vi "Setup UI.vi"(8 "error in (no error)":errorcluster, 10 "Set UI to input? (F)":bool, 11 "Pulse Gen Scan in":refnum<class "Pulse Gen Scan.lvclass">) -> (0 "error out":errorcluster, 3 "Pulse Gen Scan out":refnum<class "Pulse Gen Scan.lvclass">)   [LabVIEW 2015, in "Pulse Gen Scan.lvclass"]
doc: "Scanner::Setup is a constructor that has no parameters and faces the user. The Factory calls this VI to let the user configure this Scanner. It is dynamically dispatched in order to let the user choose the type as well as the options of the scanner."
uses:
  Pulse Gen Scan.lvclass
  Pulse Gen Scan.lvclass/Pulse Gen Scan.ctl
panel:
  in  "Gated":bool
  in  "Switch Ch1 and Ch2 Outputs":bool
  in  "template: seperate \nch 1 pump/ ch2 probe":bool
  in  "Width/Dutycycle\nUP/Down":bool
  in  "dutycycle3":dbl
  in  "dutycycle2":dbl
  in  "dutycycle1":dbl
  out "Expected external period/frequency (text)":string="Expected external period/frequency"
  out "Desired overall period/frequency (text)":string="Desired overall period/frequency"
  in  "Trigger Mode":bool caption="External"
  in  "template: Rabi scan":bool
  out "Array of Ch2 times used":dbl[unit][](array[numeric])
  in  "Repeat sequence,\ncentered on 3T/4?":bool
  in  "Ch1 pulses centered \non trigger T/4?":enum32{"none", "first", "second"}(radio)
  out "time per bit":dbl[unit]
  out "Array of Ch1 times used":dbl[unit][](array[numeric])
  in  "period/frequency":bool
  in  "template: spin echo scan":bool
  in  "template: pump/probe scan":bool
  in  "template: pulse width scan":bool
  in  "indCh2width?":bool
  in  "indChdelay?":bool
  in  "indWidth3?":bool
  in  "indDelay3?":bool
  in  "ind3Width2?":bool
  in  "indDelay2?":bool
  in  "indWidth1?":bool
  in  "indDelay1?":bool
  in  "Overall frequency":dbl[unit]
  in  "Overall period":dbl[unit]
  in  "Ch2width":dbl[unit]
  in  "Ch2delay":dbl[unit]
  in  "width3":dbl[unit]
  in  "delay3":dbl[unit]
  in  "width2":dbl[unit]
  in  "delay2":dbl[unit]
  in  "width1":dbl[unit]
  in  "delay1":dbl[unit]
  in  "Send conds for first point to PG":bool
  out "Ch 1 Digital Waveform Graph":digitalwaveform(graph)
  out "Ch1 output string":string
  out "Ch2 output string":string
  out "Ch 2 Digital Waveform Graph":digitalwaveform(graph)
  in  "Ch2 Delay relative \nto end of Ch1?":bool
  # "ind. variable?"
  # "PURE VIRTUAL\nMETHOD CALLED!"
  # "Internal"
  # "Pulse Gen Scan"
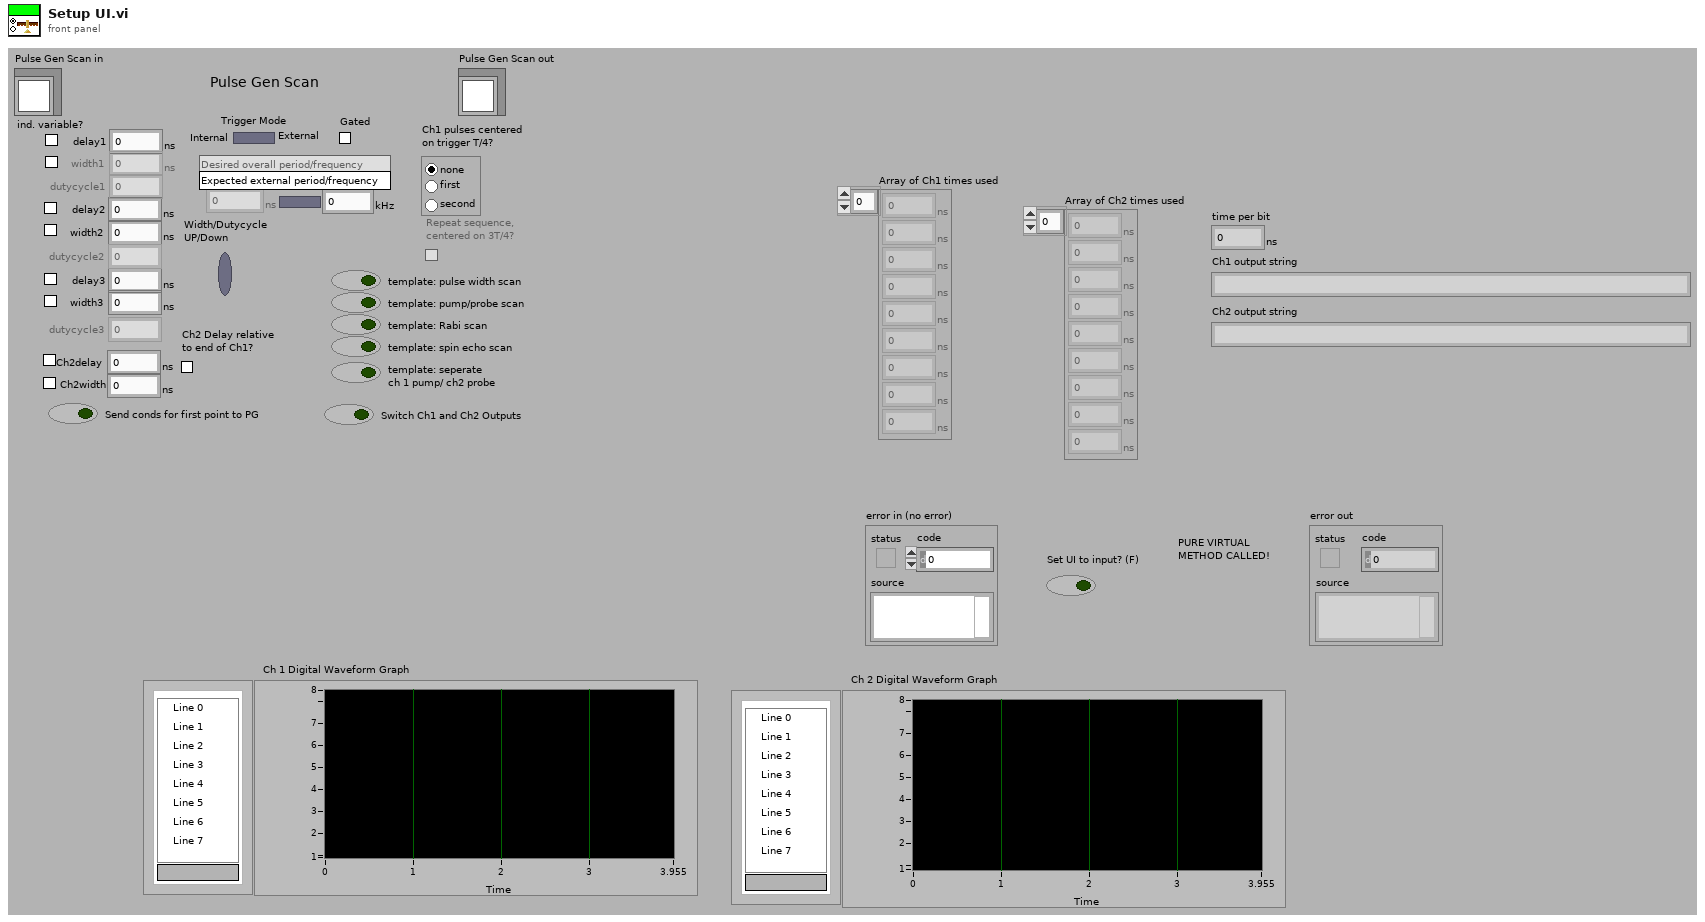
[diagram p1: front panel]
types:
  T1 = typedef "Scanner.lvclass/Range.ctl" = cluster{"xi":dbl, "xf":dbl, "dx":dbl, "Return to...?":bool, "Return to":dbl}
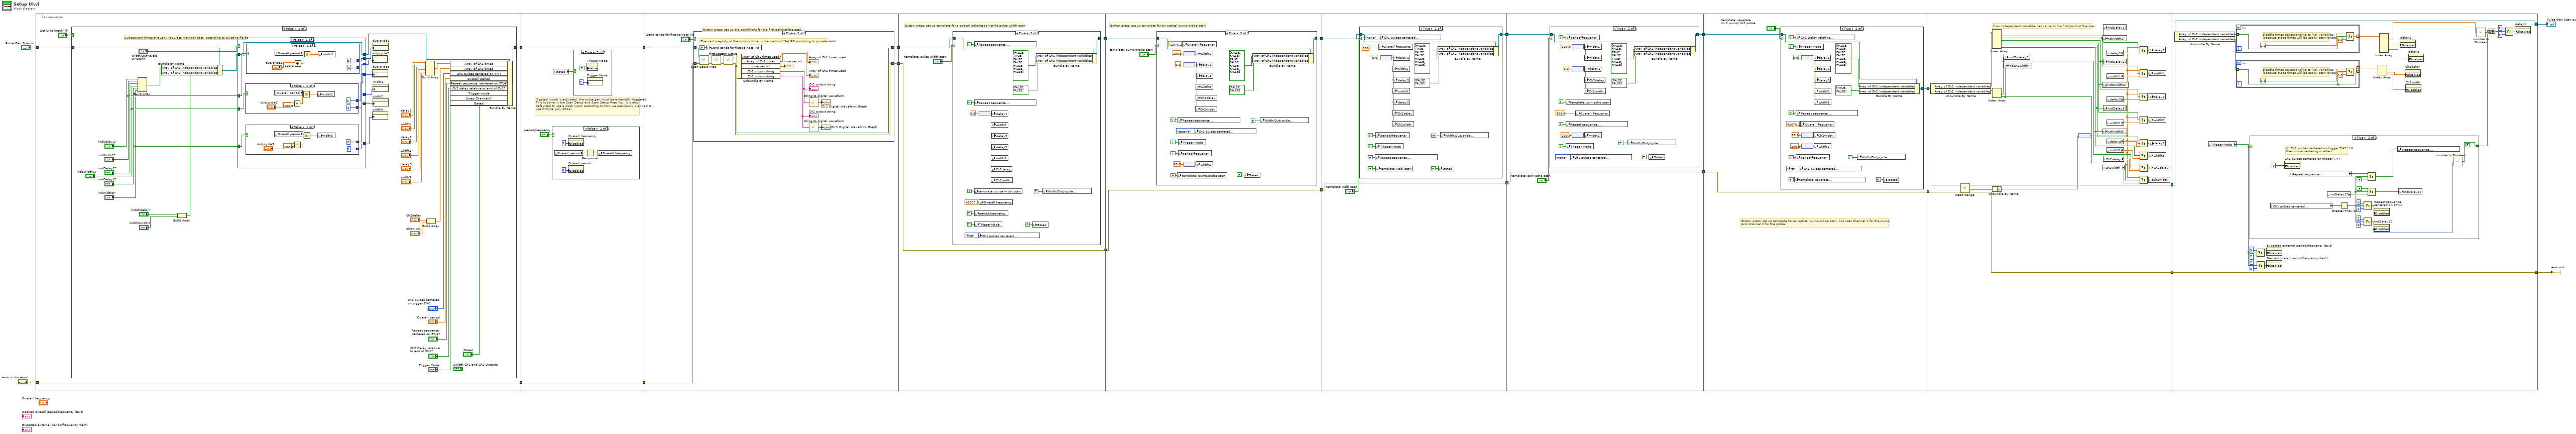
[diagram p0: block diagram]
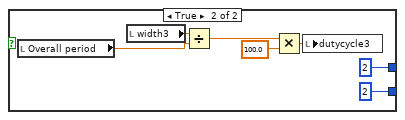
[diagram p2: hidden frame]
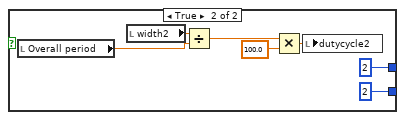
[diagram p3: hidden frame]
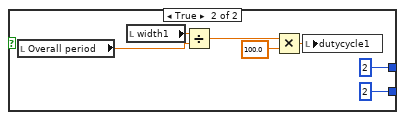
[diagram p4: hidden frame]
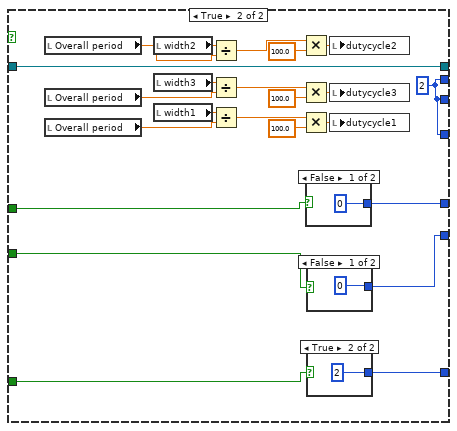
[diagram p5: hidden frame]
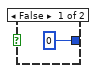
[diagram p6: hidden frame]
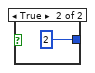
[diagram p7: hidden frame]
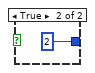
[diagram p8: hidden frame]
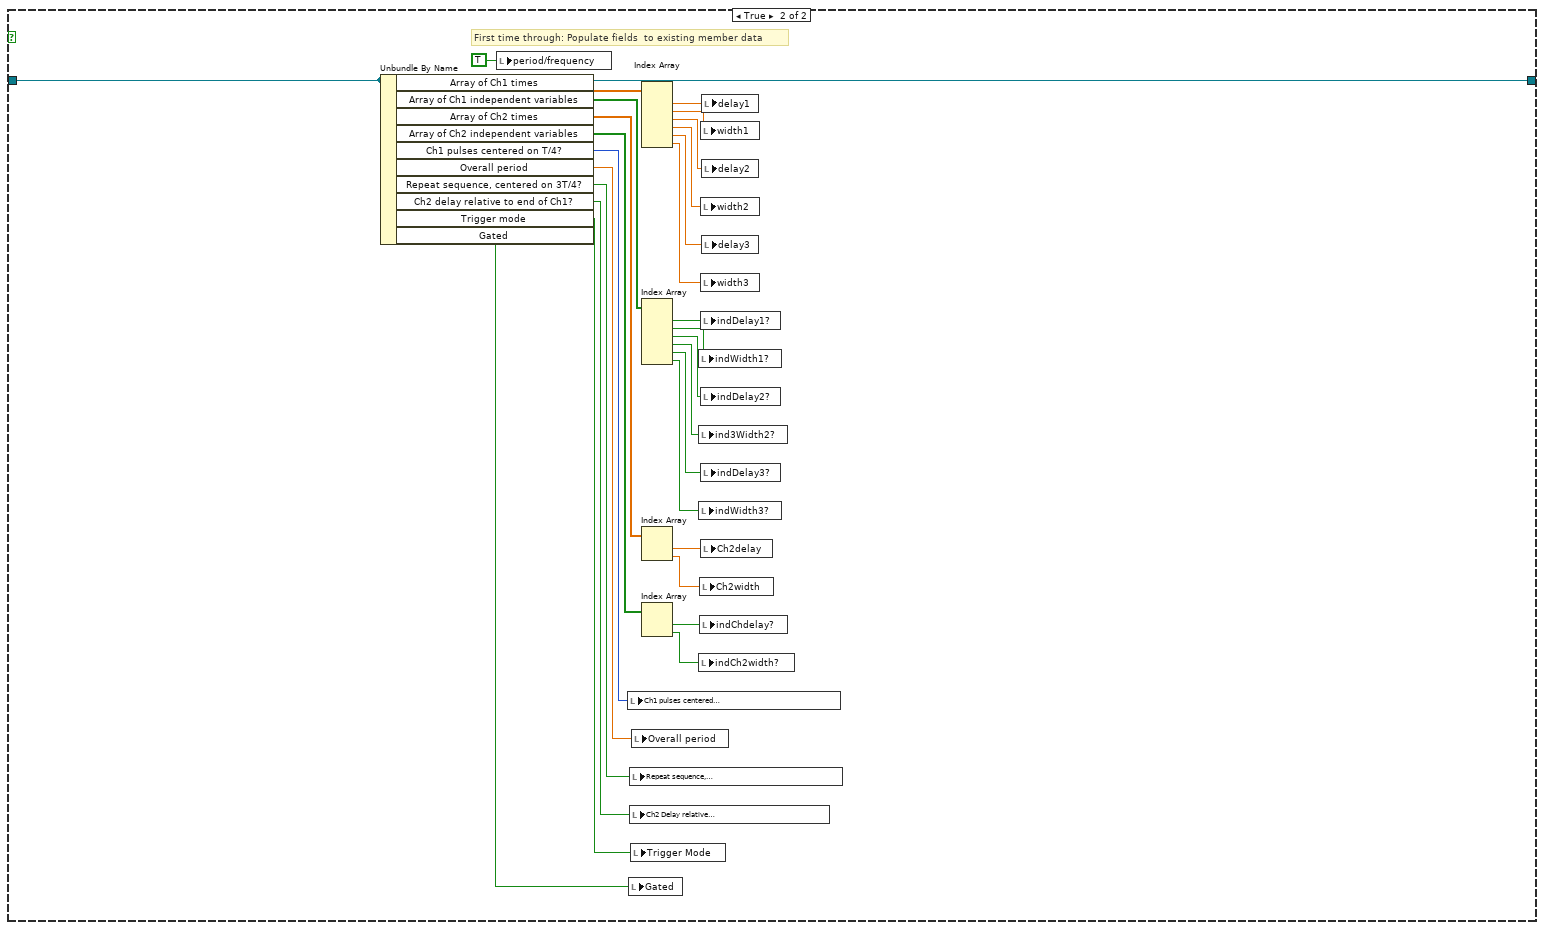
[diagram p9: hidden frame]
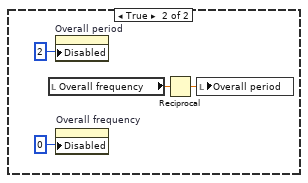
[diagram p10: hidden frame]
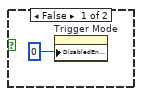
[diagram p11: hidden frame]
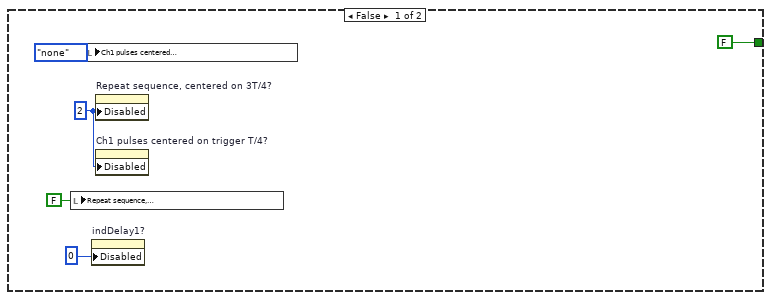
[diagram p18: hidden frame]
diagram:
  n1 = flat-sequence {
    tunnel: "error in (no error)" -> [w24]
    tunnel: "Pulse Gen Scan in" -> [w25]
    tunnel: [w23] -> w6
    tunnel: [w24] -> w4
    tunnel: w6 -> [w177]
    tunnel: [w177] -> w5
    tunnel: w4 -> [w176]
    tunnel: [w176] -> w3
    tunnel: w5 -> [w193]
    tunnel: [w191] -> w18
    tunnel: w3 -> [w192]
    tunnel: [w190] -> w17
    tunnel: w18 -> [w213]
    tunnel: [w214] -> w22
    tunnel: [w212] -> w21
    tunnel: w17 -> [w214]
    tunnel: [w232] -> w15
    tunnel: [w234] -> w13
    tunnel: w22 -> [w234]
    tunnel: w21 -> [w233]
    tunnel: w15 -> [w257]
    tunnel: [w256] -> w14
    tunnel: w13 -> [w258]
    tunnel: [w258] -> w12
    tunnel: w14 -> [w275]
    tunnel: [w274] -> w8
    tunnel: w12 -> [w276]
    tunnel: [w276] -> w7
    tunnel: w8 -> [w299]
    tunnel: w7 -> [w300]
    tunnel: [w300] -> w1
    tunnel: [w298] -> w2
    tunnel: w2 -> [w353]
    tunnel: [w352] -> w11
    tunnel: w1 -> [w351]
    tunnel: [w350] -> w10
    tunnel: w11 -> [w355]
    tunnel: w10 -> [w356]
    tunnel: [w356] -> w16
    tunnel: [w355] -> w9
    frame #0 {
      n2 = case shown="False" "Set UI to input? (F)" {
        tunnel: w25 -> [w27 w149]
        tunnel: [w46 w149] -> w23
        frame False {
          # "Subsequent times through: Populate member data  according to existing fields"
          n3 = Build Array("indDelay1?", "indWidth1?", "indDelay2?", "ind3Width2?", "indDelay3?", "indWidth3?") -> (w31:bool[])
          n4 = Build Array("indChdelay?", "indCh2width?") -> (w30:bool[])
          n5 = Bundle By Name(cluster=w27, "Array of Ch1 independent variables"=w31, "Array of Ch2 independent variables"=w30) -> (w41:refnum<class "Pulse Gen Scan.lvclass">)
          n6 = case shown="False" "Width/Dutycycle\nUP/Down" {
            tunnel: w41 -> [w65 w139]
            tunnel: [w65 w139] -> w29
            tunnel: [w68 w123] -> w40
            tunnel: [w70 w123] -> w39
            tunnel: [w72 w123] -> w38
            tunnel: "indWidth1?" -> [w74 w122]
            tunnel: "ind3Width2?" -> [w67 w121]
            tunnel: "indWidth3?" -> [w66 w120]
            tunnel: [w73 w119] -> w34
            tunnel: [w71 w117] -> w33
            tunnel: [w69 w118] -> w32
            frame False {
              n7 = case shown="False" w67 {
                tunnel: [0 2] -> w70
                tunnel: [2 2] -> w71
                frame False {
                  n8 = local read "Overall period"() -> (w93:dbl[unit])
                  n9 = Divide(x="dutycycle2", y=100.0) -> (x/y=w94:dbl)
                  n10 = Multiply(x=w93, y=w94) -> (x*y=w95:dbl[unit])
                  n11 = local write "width2"(w95) -> ()
                }
                frame True {
                  n12 = local read "Overall period"() -> (w98:dbl[unit])
                  n13 = local read "width2"() -> (w99:dbl[unit])
                  n14 = Divide(x=w99, y=w98) -> (x/y=w100:dbl)
                  n15 = Multiply(x=w100, y=100.0) -> (x*y=w102:dbl)
                  n16 = local write "dutycycle2"(w102) -> ()
                }
              }
              n17 = case shown="False" w66 {
                tunnel: [0 2] -> w72
                tunnel: [2 2] -> w73
                frame False {
                  n18 = local read "Overall period"() -> (w79:dbl[unit])
                  n19 = Divide(x="dutycycle3", y=100.0) -> (x/y=w80:dbl)
                  n20 = Multiply(x=w79, y=w80) -> (x*y=w81:dbl[unit])
                  n21 = local write "width3"(w81) -> ()
                }
                frame True {
                  n22 = local read "Overall period"() -> (w84:dbl[unit])
                  n23 = local read "width3"() -> (w85:dbl[unit])
                  n24 = Divide(x=w85, y=w84) -> (x/y=w86:dbl)
                  n25 = Multiply(x=w86, y=100.0) -> (x*y=w88:dbl)
                  n26 = local write "dutycycle3"(w88) -> ()
                }
              }
              n27 = case shown="False" w74 {
                tunnel: [0 2] -> w68
                tunnel: [2 2] -> w69
                frame False {
                  n28 = local read "Overall period"() -> (w107:dbl[unit])
                  n29 = Divide(x="dutycycle1", y=100.0) -> (x/y=w108:dbl)
                  n30 = Multiply(x=w107, y=w108) -> (x*y=w109:dbl[unit])
                  n31 = local write "width1"(w109) -> ()
                }
                frame True {
                  n32 = local read "Overall period"() -> (w112:dbl[unit])
                  n33 = local read "width1"() -> (w113:dbl[unit])
                  n34 = Divide(x=w113, y=w112) -> (x/y=w114:dbl)
                  n35 = Multiply(x=w114, y=100.0) -> (x*y=w116:dbl)
                  n36 = local write "dutycycle1"(w116) -> ()
                }
              }
            }
            frame True {
              w123 = 2
              n37 = local read "Overall period"() -> (w137:dbl[unit])
              n38 = local read "Overall period"() -> (w136:dbl[unit])
              n39 = local read "Overall period"() -> (w138:dbl[unit])
              n40 = local read "width2"() -> (w134:dbl[unit])
              n41 = local read "width3"() -> (w135:dbl[unit])
              n42 = local read "width1"() -> (w133:dbl[unit])
              n43 = Divide(x=w134, y=w137) -> (x/y=w131:dbl)
              n44 = Divide(x=w135, y=w136) -> (x/y=w130:dbl)
              n45 = Divide(x=w133, y=w138) -> (x/y=w132:dbl)
              n46 = Multiply(x=w131, y=100.0) -> (x*y=w125:dbl)
              n47 = Multiply(x=w130, y=100.0) -> (x*y=w126:dbl)
              n48 = Multiply(x=w132, y=100.0) -> (x*y=w124:dbl)
              n49 = case shown="False" w122 {
                tunnel: [0 2] -> w118
                frame False {
                }
                frame True {
                }
              }
              n50 = case shown="False" w121 {
                tunnel: [0 2] -> w117
                frame False {
                }
                frame True {
                }
              }
              n51 = case shown="True" w120 {
                tunnel: [0 2] -> w119
                frame False {
                }
                frame True {
                }
              }
              n52 = local write "dutycycle2"(w125) -> ()
              n53 = local write "dutycycle3"(w126) -> ()
              n54 = local write "dutycycle1"(w124) -> ()
            }
          }
          n55 = property on="dutycycle2" class="DigNum (strict)"("DisabledEnum"=w39) -> ()  [unwired: 2 in, 2 out]
          n56 = property on="dutycycle3" class="DigNum (strict)"("DisabledEnum"=w38) -> ()  [unwired: 2 in, 2 out]
          n57 = property on="width3" class="DigNum (strict)"("DisabledEnum"=w34) -> ()  [unwired: 2 in, 2 out]
          n58 = property on="dutycycle1" class="DigNum (strict)"("DisabledEnum"=w40) -> ()  [unwired: 2 in, 2 out]
          n59 = property on="width2" class="DigNum (strict)"("DisabledEnum"=w33) -> ()  [unwired: 2 in, 2 out]
          n60 = property on="width1" class="DigNum (strict)"("DisabledEnum"=w32) -> ()  [unwired: 2 in, 2 out]
          n61 = Build Array("delay1", "width1", "delay2", "width2", "delay3", "width3") -> (w28:dbl[unit][])
          n62 = Build Array("Ch2delay", "Ch2width") -> (w51:dbl[unit][])
          n63 = Bundle By Name(cluster=w29, "Array of Ch1 times"=w28, "Array of Ch2 times"=w51, "Ch1 pulses centered on T/4?"="Ch1 pulses centered \non trigger T/4?", "Overall period"="Overall period", "Repeat sequence, centered on 3T/4?"="Repeat sequence,\ncentered on 3T/4?", "Ch2 delay relative to end of Ch1?"="Ch2 Delay relative \nto end of Ch1?", "Trigger mode"="Trigger Mode", "Swap Channels?"="Switch Ch1 and Ch2 Outputs", "Gated"="Gated") -> (w46:refnum<class "Pulse Gen Scan.lvclass">)
        }
        frame True {
          # "First time through: Populate fields  to existing member data"
          n64 = Unbundle By Name(w149) -> ("Array of Ch1 times"=w161:dbl[unit][], "Array of Ch1 independent variables"=w155:bool[], "Array of Ch2 times"=w160:dbl[unit][], "Array of Ch2 independent variables"=w154:bool[], "Ch1 pulses centered on T/4?"=w152:enum32{"none", "first", "second"}, "Overall period"=w153:dbl[unit], "Repeat sequence, centered on 3T/4?"=w151:bool, "Ch2 delay relative to end of Ch1?"=w150:bool, "Trigger mode"=w148:bool, "Gated"=w146:bool)
          n65 = local write "period/frequency"(TRUE) -> ()
          n66 = local write "Ch1 pulses centered \non trigger T/4?"(w152) -> ()
          n67 = local write "Gated"(w146) -> ()
          n68 = local write "Repeat sequence,\ncentered on 3T/4?"(w151) -> ()
          n69 = local write "Ch2 Delay relative \nto end of Ch1?"(w150) -> ()
          n70 = local write "Trigger Mode"(w148) -> ()
          n71 = local write "Overall period"(w153) -> ()
          n72 = Index Array(array=w161) -> (element #1=w173:dbl[unit], element #2=w172:dbl[unit], element #3=w171:dbl[unit], element #4=w170:dbl[unit], element #5=w169:dbl[unit], element #6=w168:dbl[unit])  [unwired: 6 in]
          n73 = Index Array(array=w155) -> (element #1=w162:bool, element #2=w163:bool, element #3=w164:bool, element #4=w165:bool, element #5=w166:bool, element #6=w147:bool)  [unwired: 6 in]
          n74 = Index Array(array=w160) -> (element #1=w159:dbl[unit], element #2=w158:dbl[unit])  [unwired: 2 in]
          n75 = Index Array(array=w154) -> (element #1=w157:bool, element #2=w156:bool)  [unwired: 2 in]
          n76 = local write "indWidth1?"(w163) -> ()
          n77 = local write "ind3Width2?"(w165) -> ()
          n78 = local write "indWidth3?"(w147) -> ()
          n79 = local write "indCh2width?"(w156) -> ()
          n80 = local write "Ch2width"(w158) -> ()
          n81 = local write "indChdelay?"(w157) -> ()
          n82 = local write "width1"(w172) -> ()
          n83 = local write "width2"(w170) -> ()
          n84 = local write "width3"(w168) -> ()
          n85 = local write "indDelay1?"(w162) -> ()
          n86 = local write "indDelay2?"(w164) -> ()
          n87 = local write "indDelay3?"(w166) -> ()
          n88 = local write "Ch2delay"(w159) -> ()
          n89 = local write "delay1"(w173) -> ()
          n90 = local write "delay2"(w171) -> ()
          n91 = local write "delay3"(w169) -> ()
        }
      }
    }
    frame #1 {
      # "If gated mode is activated, the pulse gen must be externally triggered.  This is done in the Scan Setup and Scan Setup Prep VIs.  It is also defaulted to use a clock input, according to how we previously planned to use it (Kyle, July 2014)"
      n92 = case shown="False" "period/frequency" {
        frame False {
          n93 = local read "Overall period"() -> (w178:dbl[unit])
          n94 = property on="Overall frequency" class="DigNum (strict)"("Disabled"=2 ("f")) -> ()  [unwired: 2 in, 2 out]
          n95 = property on="Overall period" class="DigNum (strict)"("Disabled"=0) -> ()  [unwired: 2 in, 2 out]
          n96 = Reciprocal(x=w178) -> (1/x=w179:dbl[unit])
          n97 = local write "Overall frequency"(w179) -> ()
        }
        frame True {
          n98 = local read "Overall frequency"() -> (w183:dbl[unit])
          n99 = property on="Overall period" class="DigNum (strict)"("Disabled"=2) -> ()  [unwired: 2 in, 2 out]
          n100 = property on="Overall frequency" class="DigNum (strict)"("Disabled"=0 ("f")) -> ()  [unwired: 2 in, 2 out]
          n101 = Reciprocal(x=w183) -> (1/x=w182:dbl[unit])
          n102 = local write "Overall period"(w182) -> ()
        }
      }
      n103 = local read "Gated"() -> (w175:bool)
      n104 = case shown="True" w175 {
        frame False {
          n105 = property on="Trigger Mode" class="Bool (strict)"("DisabledEnum"=0) -> ()  [unwired: 2 in, 2 out]
        }
        frame True {
          n106 = property on="Trigger Mode" class="Bool (strict)"("Value"=TRUE ("Trigger Mode")) -> ()  [unwired: 2 in, 2 out]
          n107 = property on="Trigger Mode" class="Bool (strict)"("DisabledEnum"=2) -> ()  [unwired: 2 in, 2 out]
        }
      }
    }
    frame #2 {
      # "Button press: set up the conditions for the first point of the scan"
      n108 = case shown="True" "Send conds for first point to PG" {
        tunnel: [w195 w201] -> w191
        tunnel: [w194 w200] -> w190
        tunnel: w193 -> [w195 w197]
        tunnel: w192 -> [w194 w196]
        frame False {
        }
        frame True {
          # "The vast majority of the work is done in the method \"Set PG according to private data\""
          n109 = call "Scan Setup Prep.vi"("error in (no error)"=w196, "Pulse Gen Scan in"=w197) -> ("error out"=w199:errorcluster, "Pulse Gen Scan out"=w198:refnum<class "Pulse Gen Scan.lvclass">)  [unwired: 8 in]
          n110 = local write "Send conds for first point to PG"(FALSE ("Send conds for first point to PG")) -> ()
          n111 = call-dynamic "First Step.vi"("error in (no error)"=w199, "Pulse Gen Scan.lvclass in"=w198) -> ("error out"=w202:errorcluster, "Pulse Gen Scan.lvclass out"=w203:refnum<class "Pulse Gen Scan.lvclass">)  [unwired: 8 out]
          n112 = call-dynamic "Scan Setup.vi"("error in (no error)"=w202, "Pulse Gen Scan in"=w203) -> ("error out"=w200:errorcluster, "Pulse Gen Scan out"=w201:refnum<class "Pulse Gen Scan.lvclass">)  [unwired: 8 out]
          n113 = Unbundle By Name(w201) -> ("Array of Ch1 times used"=→"Array of Ch1 times used":dbl[unit][], "Array of Ch2 times"=→"Array of Ch2 times used":dbl[unit][], "time per bit"=→"time per bit":dbl[unit], "Ch1 output string"=w208:string, "Ch2 output string"=w207:string)
          "Ch1 output string" <- w208
          "Ch2 output string" <- w207
          n114 = call "string to digital waveform.vi"("String"=w208) -> ("digital waveform"=→"Ch 1 Digital Waveform Graph":digitalwaveform)
          n115 = call "string to digital waveform.vi"("String"=w207) -> ("digital waveform"=→"Ch 2 Digital Waveform Graph":digitalwaveform)
        }
      }
    }
    frame #3 {
      # "Button press: set up template for a optical polarization-style pulse-width scan"
      n116 = case shown="True" "template: pulse width scan" {
        tunnel: w213 -> [w216 w228]
        tunnel: [w216 w227] -> w212
        frame False {
        }
        frame True {
          n117 = local write "Repeat sequence,\ncentered on 3T/4?"(TRUE ("Repeat sequence,\ncentered on 3T/4?")) -> ()
          n118 = local write "Repeat sequence,\ncentered on 3T/4?"(TRUE ("Repeat sequence,\ncentered on 3T/4?")) -> ()
          n119 = local write "template: pulse width scan"(FALSE) -> ()
          n120 = local write "period/frequency"(TRUE ("period/frequency")) -> ()
          n121 = local write "Trigger Mode"(TRUE ("Trigger Mode")) -> ()
          n122 = local write "Ch1 pulses centered \non trigger T/4?"(enum32{"none", "first", "second"}."first" ("Pulses centered \non T/4?")) -> ()
          n123 = node(0.0) -> (w219:dbl[unit])
          n124 = local write "Overall frequency"(dbl[unit] 42077.3 ("Expected frequency")) -> ()
          n125 = local write "Ch2width"(w219) -> ()
          n126 = local write "width2"(w219) -> ()
          n127 = local write "width3"(w219) -> ()
          n128 = local write "Ch2delay"(w219) -> ()
          n129 = local write "delay1"(w219) -> ()
          n130 = local write "delay3"(w219) -> ()
          n131 = local write "delay2"(w219) -> ()
          n132 = local write "Gated"(FALSE ("Gated")) -> ()
          n133 = Bundle By Name(cluster=w228, "Array of Ch1 independent variables"=bool[] [FALSE, TRUE, FALSE, FALSE, FALSE, FALSE, FALSE], "Array of Ch2 independent variables"=bool[] [FALSE, FALSE]) -> (w227:refnum<class "Pulse Gen Scan.lvclass">)
          n134 = local write "Width/Dutycycle\nUP/Down"(TRUE ("period/frequency")) -> ()
        }
      }
    }
    frame #4 {
      # "Button press: set up template for an optical pump-probe scan"
      n135 = case shown="True" "template: pump/probe scan" {
        tunnel: w233 -> [w236 w248]
        tunnel: [w236 w246] -> w232
        frame False {
        }
        frame True {
          n136 = local write "template: pump/probe scan"(FALSE) -> ()
          n137 = local write "Repeat sequence,\ncentered on 3T/4?"(TRUE ("Repeat sequence,\ncentered on 3T/4?")) -> ()
          n138 = local write "Trigger Mode"(TRUE ("Trigger Mode")) -> ()
          n139 = local write "period/frequency"(TRUE ("period/frequency")) -> ()
          n140 = local write "Overall frequency"(dbl[unit] 42076.2 ("Expected frequency")) -> ()
          n141 = node(200.0) -> (w252:dbl[unit])
          n142 = node(0.0) -> (w239:dbl[unit])
          n143 = node(50.0) -> (w254:dbl[unit])
          n144 = local write "Ch1 pulses centered \non trigger T/4?"(enum32{"none", "first", "second"}."second" ("Pulses centered \non T/4?")) -> ()
          n145 = local write "Ch2width"(w239) -> ()
          n146 = local write "width1"(w252) -> ()
          n147 = local write "width3"(w239) -> ()
          n148 = local write "Ch2delay"(w239) -> ()
          n149 = local write "width2"(w254) -> ()
          n150 = local write "delay1"(w239) -> ()
          n151 = local write "delay3"(w239) -> ()
          n152 = local write "Gated"(FALSE ("Gated")) -> ()
          n153 = Bundle By Name(cluster=w248, "Array of Ch1 independent variables"=bool[] [FALSE, FALSE, TRUE, FALSE, FALSE, FALSE, FALSE], "Array of Ch2 independent variables"=bool[] [FALSE, FALSE]) -> (w246:refnum<class "Pulse Gen Scan.lvclass">)
          n154 = local write "Width/Dutycycle\nUP/Down"(TRUE ("period/frequency")) -> ()
        }
      }
    }
    frame #5 {
      n155 = case shown="True" "template: Rabi scan" {
        tunnel: w257 -> [w259 w270]
        tunnel: [w259 w269] -> w256
        frame False {
        }
        frame True {
          n156 = local write "Repeat sequence,\ncentered on 3T/4?"(FALSE ("Repeat sequence,\ncentered on 3T/4?")) -> ()
          n157 = local write "period/frequency"(TRUE ("period/frequency")) -> ()
          n158 = local write "Trigger Mode"(TRUE ("Trigger Mode")) -> ()
          n159 = local write "template: Rabi scan"(FALSE) -> ()
          n160 = local write "Overall frequency"(dbl[unit] 200000.0 ("Expected frequency")) -> ()
          n161 = local write "Ch1 pulses centered \non trigger T/4?"(enum32{"none", "first", "second"}."none" ("Pulses centered \non T/4?")) -> ()
          n162 = node(0.0) -> (w264:dbl[unit])
          n163 = local write "Ch2width"(w264) -> ()
          n164 = local write "width2"(w264) -> ()
          n165 = local write "width3"(w264) -> ()
          n166 = local write "Ch2delay"(w264) -> ()
          n167 = local write "delay1"(w264) -> ()
          n168 = local write "delay3"(w264) -> ()
          n169 = local write "delay2"(w264) -> ()
          n170 = Bundle By Name(cluster=w270, "Array of Ch1 independent variables"=bool[] [FALSE, TRUE, FALSE, FALSE, FALSE, FALSE, FALSE], "Array of Ch2 independent variables"=bool[] [FALSE, FALSE]) -> (w269:refnum<class "Pulse Gen Scan.lvclass">)
          n171 = local write "Gated"(FALSE ("Gated")) -> ()
          n172 = local write "Width/Dutycycle\nUP/Down"(TRUE ("period/frequency")) -> ()
        }
      }
    }
    frame #6 {
      n173 = case shown="True" "template: spin echo scan" {
        tunnel: w275 -> [w278 w289]
        tunnel: [w278 w287] -> w274
        frame False {
        }
        frame True {
          n174 = local write "template: spin echo scan"(FALSE) -> ()
          n175 = local write "Repeat sequence,\ncentered on 3T/4?"(FALSE ("Repeat sequence,\ncentered on 3T/4?")) -> ()
          n176 = local write "period/frequency"(TRUE ("period/frequency")) -> ()
          n177 = local write "Trigger Mode"(TRUE ("Trigger Mode")) -> ()
          n178 = local write "Ch1 pulses centered \non trigger T/4?"(enum32{"none", "first", "second"}."none" ("Pulses centered \non T/4?")) -> ()
          n179 = node(100.0) -> (w296:dbl[unit])
          n180 = node(0.0) -> (w292:dbl[unit])
          n181 = node(200.0) -> (w295:dbl[unit])
          n182 = local write "Overall frequency"(dbl[unit] 900.0 ("Expected frequency")) -> ()
          n183 = local write "Ch2width"(w292) -> ()
          n184 = local write "width1"(w296) -> ()
          n185 = local write "width3"(w296) -> ()
          n186 = local write "Ch2delay"(w292) -> ()
          n187 = local write "width2"(w295) -> ()
          n188 = local write "delay1"(w292) -> ()
          n189 = local write "Width/Dutycycle\nUP/Down"(TRUE ("period/frequency")) -> ()
          n190 = Bundle By Name(cluster=w289, "Array of Ch1 independent variables"=bool[] [FALSE, FALSE, TRUE, FALSE, TRUE, FALSE, FALSE], "Array of Ch2 independent variables"=bool[] [FALSE, FALSE]) -> (w287:refnum<class "Pulse Gen Scan.lvclass">)
          n191 = local write "Gated"(TRUE ("Gated")) -> ()
        }
      }
    }
    frame #7 {
      # "Button press: set up template for an optical pump-probe scan, but uses channel 1 for the pump\nand channel 2 for the probe."
      n192 = case shown="True" "template: seperate \nch 1 pump/ ch2 probe" {
        tunnel: w299 -> [w301 w318]
        tunnel: [w301 w317] -> w298
        frame False {
        }
        frame True {
          n193 = local write "template: seperate \nch 1 pump/ ch2 probe"(FALSE) -> ()
          n194 = local write "Ch2 Delay relative \nto end of Ch1?"(TRUE ("period/frequency")) -> ()
          n195 = local write "Repeat sequence,\ncentered on 3T/4?"(TRUE ("Trigger Mode")) -> ()
          n196 = local write "Trigger Mode"(TRUE ("Trigger Mode")) -> ()
          n197 = local write "period/frequency"(TRUE ("Trigger Mode")) -> ()
          n198 = local write "Ch1 pulses centered \non trigger T/4?"(enum32{"none", "first", "second"}."first" ("Pulses centered \non T/4?")) -> ()
          n199 = local write "Overall frequency"(dbl[unit] 42076.2 ("Expected frequency")) -> ()
          n200 = node(0.0) -> (w306:dbl[unit])
          n201 = node(50.0) -> (w316:dbl[unit])
          n202 = node(200.0) -> (w314:dbl[unit])
          n203 = local write "Ch2width"(w316) -> ()
          n204 = local write "width2"(w306) -> ()
          n205 = local write "width3"(w306) -> ()
          n206 = local write "width1"(w314) -> ()
          n207 = local write "delay1"(w306) -> ()
          n208 = local write "delay2"(w306) -> ()
          n209 = local write "delay3"(w306) -> ()
          n210 = local write "Width/Dutycycle\nUP/Down"(TRUE ("period/frequency")) -> ()
          n211 = Bundle By Name(cluster=w318, "Array of Ch1 independent variables"=bool[] [FALSE, FALSE, FALSE, FALSE, FALSE, FALSE, FALSE], "Array of Ch2 independent variables"=bool[] [TRUE, FALSE]) -> (w317:refnum<class "Pulse Gen Scan.lvclass">)
          n212 = local write "Gated"(FALSE ("Gated")) -> ()
        }
      }
    }
    frame #8 {
      # "If an independent variable, set value to the first point of the scan"
      n213 = Unbundle By Name(w353) -> ("Array of Ch1 independent variables"=w324:bool[], "Array of Ch2 independent variables"=w323:bool[])
      n214 = call-dynamic "Read Range.vi"("error in (no error)"=w351, "Scanner.lvclass in"=w353) -> ("error out"=w350:errorcluster, "Range"=w349:T1, "Scanner.lvclass out"=w352:refnum<class "Pulse Gen Scan.lvclass">)  [unwired: 7 out]
      n215 = Index Array(array=w324) -> (element #1=w325:bool, element #2=w342:bool, element #3=w343:bool, element #4=w344:bool, element #5=w345:bool, element #6=w346:bool)  [unwired: 6 in]
      n216 = Index Array(array=w323) -> (element #1=w347:bool, element #2=w348:bool)  [unwired: 2 in]
      n217 = Unbundle By Name(w349) -> ("xi"=w321:dbl)
      n218 = local write "indCh2width?"(w348) -> ()
      n219 = local write "indChdelay?"(w347) -> ()
      n220 = node(w321) -> (w322:dbl[unit])
      n221 = local write "indWidth1?"(w342) -> ()
      n222 = local write "ind3Width2?"(w344) -> ()
      n223 = local write "indWidth3?"(w346) -> ()
      n224 = local read "Ch2width"() -> (w340:dbl[unit])
      n225 = local write "indDelay1?"(w325) -> ()
      n226 = local write "indDelay2?"(w343) -> ()
      n227 = local write "indDelay3?"(w345) -> ()
      n228 = local read "Ch2delay"() -> (w339:dbl[unit])
      n229 = local read "width1"() -> (w328:dbl[unit])
      n230 = local read "width2"() -> (w332:dbl[unit])
      n231 = local read "width3"() -> (w336:dbl[unit])
      n232 = local read "delay1"() -> (w327:dbl[unit])
      n233 = local read "delay2"() -> (w331:dbl[unit])
      n234 = local read "delay3"() -> (w335:dbl[unit])
      n235 = Select(t=w322, s=w325, f=w327) -> (s? t:f=w326:dbl[unit])
      n236 = Select(t=w322, s=w342, f=w328) -> (s? t:f=w329:dbl[unit])
      n237 = Select(t=w322, s=w343, f=w331) -> (s? t:f=w330:dbl[unit])
      n238 = Select(t=w322, s=w344, f=w332) -> (s? t:f=w333:dbl[unit])
      n239 = Select(t=w322, s=w345, f=w335) -> (s? t:f=w334:dbl[unit])
      n240 = Select(t=w322, s=w346, f=w336) -> (s? t:f=w337:dbl[unit])
      n241 = Select(t=w322, s=w347, f=w339) -> (s? t:f=w338:dbl[unit])
      n242 = Select(t=w322, s=w348, f=w340) -> (s? t:f=w341:dbl[unit])
      n243 = local write "Ch2width"(w341) -> ()
      n244 = local write "width1"(w329) -> ()
      n245 = local write "width2"(w333) -> ()
      n246 = local write "width3"(w337) -> ()
      n247 = local write "Ch2delay"(w338) -> ()
      n248 = local write "delay1"(w326) -> ()
      n249 = local write "delay2"(w330) -> ()
      n250 = local write "delay3"(w334) -> ()
    }
    frame #9 {
      n251 = Unbundle By Name(w355) -> ("Array of Ch1 independent variables"=w354:bool[], "Array of Ch2 independent variables"=w373:bool[])
      n252 = local read "Trigger Mode"() -> (w358:bool)
      n253 = for {
        tunnel: [w404] -> w377 mode=indexing
        tunnel: w354 -> [w403] mode=indexing
        # "disable times corresponding to ind. variables \n(because those times will be set by scan range)"
        n254 = Select(t=2.0, s=w403, f=0.0) -> (s? t:f=w404:dbl)
      }
      n255 = for {
        tunnel: [w399] -> _ mode=indexing
        tunnel: [w400] -> w374 mode=indexing
        tunnel: w373 -> [w399] mode=indexing
        # "disable times corresponding to ind. variables \n(because those times will be set by scan range)"
        n256 = Select(t=2.0, s=w399, f=0.0) -> (s? t:f=w400:dbl)
      }
      n257 = case shown="True" w358 {
        tunnel: [FALSE w388] -> w359
        frame False {
          w381 = i8 2
          n258 = local write "Repeat sequence,\ncentered on 3T/4?"(FALSE ("Repeat sequence,\ncentered on 3T/4?")) -> ()
          n259 = local write "Ch1 pulses centered \non trigger T/4?"(enum32{"none", "first", "second"}."none" ("Ch1 pulses centered \non trigger T/4?")) -> ()
          n260 = property on="indDelay1?" class="Bool (strict)"("Disabled"=i8 0) -> ()  [unwired: 2 in, 2 out]
          n261 = property on="Repeat sequence, centered on 3T/4?" class="Bool (strict)"("Disabled"=w381) -> ()  [unwired: 2 in, 2 out]
          n262 = property on="Ch1 pulses centered on trigger T/4?" class="RadioBtnsControl (strict)"("Disabled"=w381) -> ()  [unwired: 2 in, 2 out]
        }
        frame True {
          (unwired) FALSE
          # "if \"Ch1 pulses centered on trigger T/4?\" >0, \nthen some centering in effect"
          n263 = local read "Ch1 pulses centered \non trigger T/4?"() -> (w394:enum32{"none", "first", "second"})
          n264 = property on="Ch1 pulses centered on trigger T/4?" class="RadioBtnsControl (strict)"("Disabled"=u8 0) -> ()  [unwired: 2 in, 2 out]
          n265 = local read "Repeat sequence,\ncentered on 3T/4?"() -> (w392:bool)
          n266 = local read "indDelay1?"() -> (w389:bool)
          n267 = Greater Than 0?(x=w394) -> (x > 0?=w386:bool)
          n268 = Select(t=0, s=w386, f=2) -> (s? t:f=w395:i32)
          n269 = Select(t=2, s=w386, f=0) -> (s? t:f=w387:i32)
          n270 = Select(t=w392, s=w386, f=FALSE) -> (s? t:f=w393:bool)
          n271 = Select(t=FALSE, s=w386, f=w389) -> (s? t:f=w391:bool)
          n272 = property on="Repeat sequence,\ncentered on 3T/4?" class="Bool (strict)"("Disabled"=w395) -> ()  [unwired: 2 in, 2 out]
          n273 = property on="indDelay1?" class="Bool (strict)"("Disabled"=w387) -> ()  [unwired: 2 in, 2 out]
          n274 = local write "Repeat sequence,\ncentered on 3T/4?"(w393) -> ()
          n275 = local write "indDelay1?"(w391) -> ()
          n276 = call "number to Boolean.vi"("Numeric"=w387) -> ("Boolean"=w388:bool)
        }
      }
      n277 = Select(t=0, s=w358, f=2) -> (s? t:f=w361:i32)
      n278 = Select(t=2, s=w358, f=0) -> (s? t:f=w360:i32)
      n279 = property on="Expected external period/frequency (text)" class="Str"("Disabled"=w361) -> ()  [unwired: 2 in, 2 out]
      n280 = property on="Desired overall period/frequency (text)" class="Str"("Disabled"=w360) -> ()  [unwired: 2 in, 2 out]
      n281 = Index Array(array=w374) -> (element #1=w372:dbl, element #2=w371:dbl)  [unwired: 2 in]
      n282 = Index Array(array=w377) -> (element #1=w370:dbl, element #3=w375:dbl, element #5=w376:dbl)  [unwired: 6 in, 3 out]
      n283 = property on="delay2" class="DigNum (strict)"("Disabled"=w375) -> ()  [unwired: 2 in, 2 out]
      n284 = property on="Ch2delay" class="DigNum (strict)"("Disabled"=w372) -> ()  [unwired: 2 in, 2 out]
      n285 = property on="Ch2width" class="DigNum (strict)"("Disabled"=w371) -> ()  [unwired: 2 in, 2 out]
      n286 = property on="delay3" class="DigNum (strict)"("Disabled"=w376) -> ()  [unwired: 2 in, 2 out]
      n287 = call "number to Boolean.vi"("Numeric"=w370) -> ("Boolean"=w369:bool)
      n288 = Or(x=w359, y=w369) -> (x .or. y?=w368:bool)
      n289 = Select(t=i8 2, s=w368, f=i8 0) -> (s? t:f=w357:i8)
      n290 = property on="delay1" class="DigNum (strict)"("Disabled"=w357) -> ()  [unwired: 2 in, 2 out]
    }
  }
  "error out" <- w16
  "Pulse Gen Scan out" <- w9
